vi "DAQmx Timing (Burst Export Clock).vi"(0 "task/channels in":refnum<k21>, 1 "sample mode":i32(ring)=10178 items=["Finite Samples"=10178, "Continuous Samples"=10123, "Hardware Timed Single Point"=12522], 2 "samples per channel":i32=1000, 5 "sample clock rate":dbl=1000.0, 7 "sample clock output terminal":tag, 9 "sample clock pulse polarity":i32(ring)=10095 items=["Active High"=10095, "Active Low"=10096], 11 "error in":errorcluster, 12 "pause when":i32(ring)=10192 items=["High"=10192, "Low"=10214], 13 "ready for transfer event active level":i32(ring)=10095 items=["Active High"=10095, "Active Low"=10096]) -> (4 "task out":refnum<k21>, 15 "error out":errorcluster)   [LabVIEW 2011]
doc: "Configures when the DAQ device transfers data to a peripheral device, using the onboard Sample Clock of the DAQ device to control burst handshake timing and exporting that clock for use by the peripheral device."
uses:
  C:/Program Files/National Instruments/LabVIEW 2011/resource/objmgr/daqmx.rc
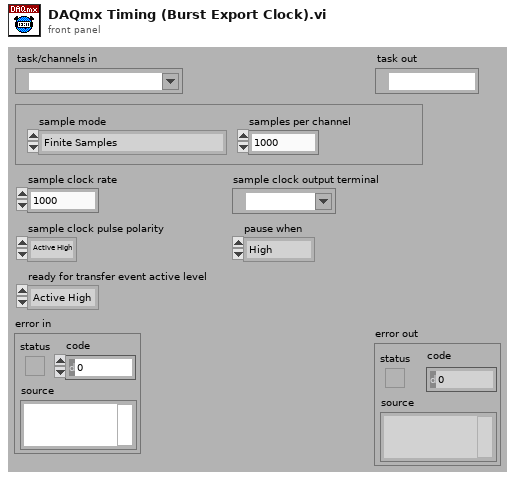
[diagram p1: front panel]
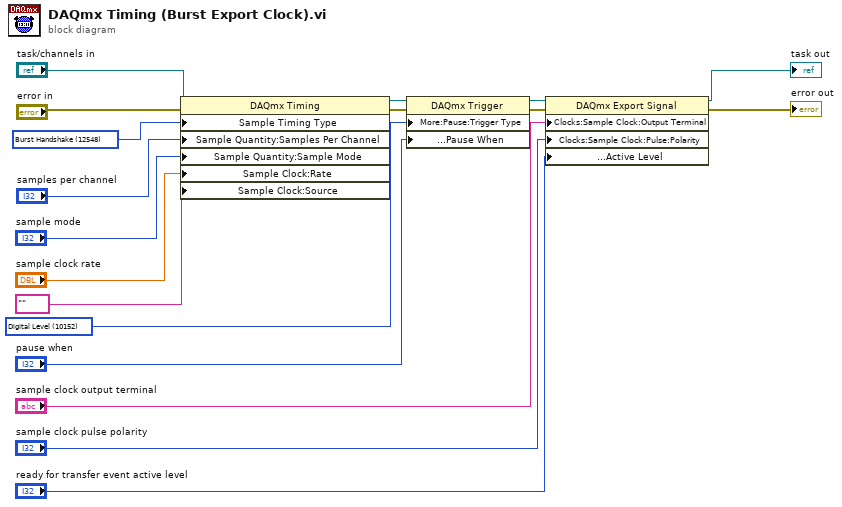
[diagram p0: block diagram]
diagram:
  w2 = 10152 items=["Analog Level"=10101, "Analog Window"=10103, "Digital Level"=10152, "None"=10230] ("Pause.TrigType")
  w14 = 12548 items=["Sample Clock"=10388, "Burst Handshake"=12548, "Handshake"=10389, "Implicit"=10451, "On Demand"=10390, "Change Detection"=12504] ("SampTimingType")
  n1 = property class="DAQmx Timing"(reference="task/channels in", error in="error in", "Sample Timing Type"=w14, "Sample Quantity:Samples Per Channel"="samples per channel", "Sample Quantity:Sample Mode"="sample mode", "Sample Clock:Rate"="sample clock rate", "Sample Clock:Source"=tag "" ("SampClk.Src")) -> (reference out=w12:refnum<k21>, error out=w11:errorcluster)
  n2 = property class="DAQmx Trigger"(reference=w12, error in=w11, "More:Pause:Trigger Type"=w2, "More:Pause:Digital Level:Pause When"="pause when") -> (reference out=w9:refnum<k21>, error out=w10:errorcluster)
  n3 = property class="DAQmx Export Signal"(reference=w9, error in=w10, "Clocks:Sample Clock:Output Terminal"="sample clock output terminal", "Clocks:Sample Clock:Pulse:Polarity"="sample clock pulse polarity", "Events:Ready For Transfer Event:Level:Active Level"="ready for transfer event active level") -> (reference out=→"task out":refnum<k21>, error out=→"error out":errorcluster)
